vi "is_done.vi"(8 "error in (no error)":errorcluster, 11 "HSDIO in":refnum<class "HSDIO.lvclass">) -> (0 "error out":errorcluster, 2 "HSDIO is done?":bool caption="done", 3 "HSDIO out":refnum<class "HSDIO.lvclass">)   [LabVIEW 2013, in "HSDIO.lvclass"]
uses:
  HSDIO.lvclass
  HSDIO.lvclass/HSDIO.ctl
  Experiment/Globals.vi
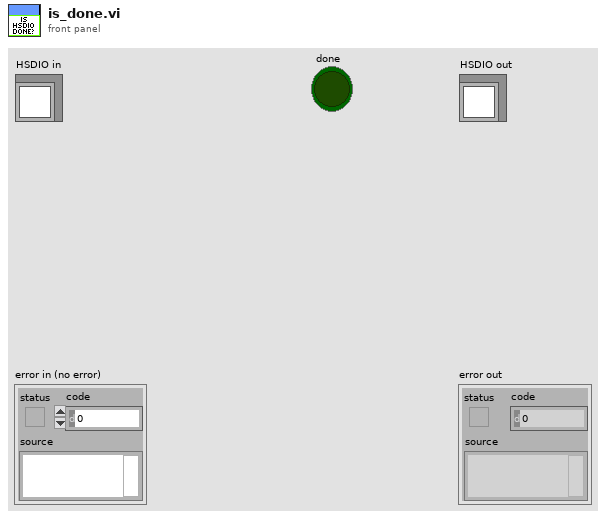
[diagram p1: front panel]
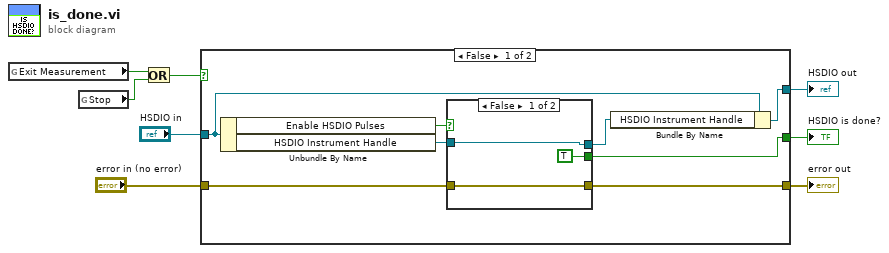
[diagram p0: block diagram]
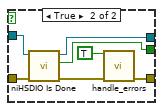
[diagram p2: hidden frame]
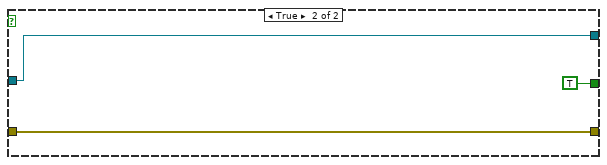
[diagram p3: hidden frame]
diagram:
  n1 = global read "Globals.vi" "Exit Measurement"() -> (w3:bool)
  n2 = global read "Globals.vi" "Stop"() -> (w4:bool)
  n3 = Or(x=w3, y=w4) -> (x .or. y?=w2:bool)
  n4 = case shown="False" w2 {
    tunnel: [w12 w28] -> w8
    tunnel: [w15 w29] -> w6
    tunnel: "HSDIO in" -> [w16 w29]
    tunnel: "error in (no error)" -> [w10 w28]
    tunnel: [w9 TRUE ("done")] -> w1
    frame False {
      n5 = Unbundle By Name(w16) -> ("Enable HSDIO Pulses"=w14:bool, "HSDIO Instrument Handle"=w13:refnum<k15>)
      n6 = case shown="False" w14 {
        tunnel: w13 -> [w19 w26]
        tunnel: w10 -> [w18 w25]
        tunnel: [w18 w21] -> w12
        tunnel: [w19 w24] -> w11
        tunnel: [TRUE ("done") w23] -> w9
        frame False {
        }
        frame True {
          n7 = call <instrlib>:"niHSDIO Is Done.vi"("error in (no error)"=w25, "instrument handle"=w26) -> ("error out"=w22:errorcluster, "done"=w23:bool, "instrument handle out"=w24:refnum<k15>)  [unwired: 7 in]
          n8 = call "handle_errors.vi"("Exit Operation"=TRUE ("Exit Measurement"), "error in (no error)"=w22) -> ("error out"=w21:errorcluster)  [unwired: 13 in]
        }
      }
      n9 = Bundle By Name(cluster=w16, "HSDIO Instrument Handle"=w11) -> (w15:refnum<class "HSDIO.lvclass">)
    }
    frame True {
    }
  }
  "error out" <- w8
  "HSDIO out" <- w6
  "HSDIO is done?" <- w1
